vi "findTransactionClicked.vi"(8 "error in (no error)":errorcluster, 10 "Coords":T1, 11 "TransactionListUserInterface in":refnum<class "TransactionListUserInterface.lvclass">) -> (0 "error out":errorcluster, 2 "Transaction.lvclass":refnum<class "Transaction.lvclass">, 3 "TransactionListUserInterface out":refnum<class "TransactionListUserInterface.lvclass">)   [LabVIEW 2018, in "TransactionListUserInterface.lvclass"]
uses:
  TransactionListUserInterface.lvclass
  <vilib>/Utility/miscctls.llb/LVPoint32TypeDef.ctl
  Transaction/Transaction.lvclass
  TransactionListUserInterface.lvclass/TransactionListUserInterface.ctl
  Banking Record/Banking Transaction.lvclass
  C:/GitRepos/Filthy-Lucre-Budgetizer/source/support/classes/Transaction/Transaction.lvclass
  Credit Record/Credit Transaction.lvclass
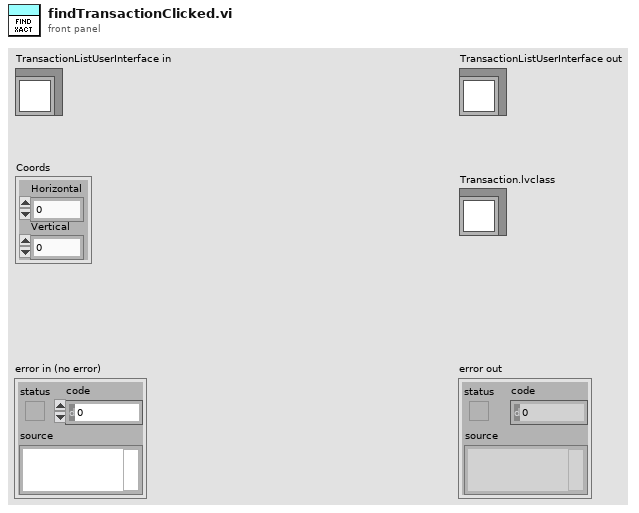
[diagram p1: front panel]
types:
  T1 = typedef "LVPoint32TypeDef.ctl" = cluster{"Horizontal":i32, "Vertical":i32}
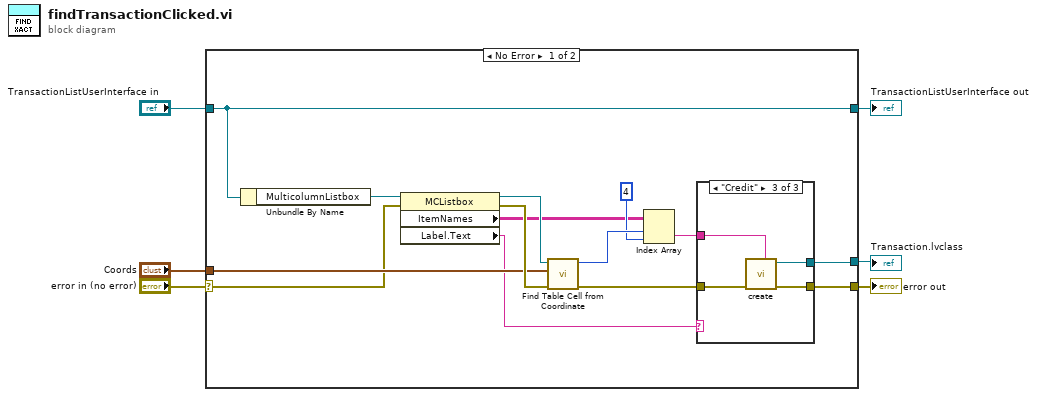
[diagram p0: block diagram]
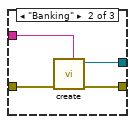
[diagram p3: hidden frame]
diagram:
  n1 = case shown="No Error" "error in (no error)" {
    selector: "error in (no error)" -> [w14 w31]
    tunnel: [w10 w31] -> w5
    tunnel: [w13 w30] -> w3
    tunnel: "TransactionListUserInterface in" -> [w13 w30]
    tunnel: "Coords" -> [w15 _]
    tunnel: [w9 _] -> w1
    frame No Error {
      n2 = Unbundle By Name(w13) -> ("MulticolumnListbox"=w12:refnum<vi>)
      n3 = property class="MCListbox"(reference=w12, error in=w14) -> (reference out=w20:refnum<vi>, error out=w19:errorcluster, "ItemNames"=w16:string[][], "Label.Text"=w8:string)
      n4 = call "Find Table Cell from Coordinate.vi"("error in (no error)"=w19, "Coords"=w15, "MCLB Refs"=w20) -> ("error out"=w11:errorcluster, "Row"=w18:u32)  [unwired: 5 in, 2 out]
      n5 = Index Array(array=w16, index (row)=w18, index (col)=4 ("disabled index (col)")) -> (element=w7:string)
      n6 = case shown="\"Credit\"" w8 {
        tunnel: w11 -> [w21 w25 w28]
        tunnel: [w21 w24 w27] -> w10
        tunnel: [_ w23 w26] -> w9
        tunnel: w7 -> [_ w22 w29]
        frame Default {
        }
        frame "Banking" {
          n7 = call "create.vi"("Reference"=w22, "error in (no error)"=w25) -> ("error out"=w24:errorcluster, "Banking Transaction out"=w23:refnum<class "Banking Transaction.lvclass">)  [unwired: 8 in]
        }
        frame "Credit" {
          n8 = call "create.vi"("Reference"=w29, "error in (no error)"=w28) -> ("error out"=w27:errorcluster, "Credit Transaction out"=w26:refnum<class "Credit Transaction.lvclass">)  [unwired: 8 in]
        }
      }
    }
    frame Error {
    }
  }
  "error out" <- w5
  "TransactionListUserInterface out" <- w3
  "Transaction.lvclass" <- w1
